vi "workbook.search.vi"(8 "error in":errorcluster, 11 "Client in":refnum<class "Client.lvclass">) -> (0 "error out":errorcluster, 3 "Client out":refnum<class "Client.lvclass">)   [LabVIEW 2020, in "Client.lvclass"]
doc: "Searches for workbooks matching the given filters (text, label, property, asset, or run) and returns a handle list of matches."
uses:
  Client.lvclass
  Client.lvclass/Client.ctl
  client.lvlib
panel:
  out "out_count out":u32
  out "out_list out":i32
  in  "out_list":i32
  in  "asset_rid":string
  in  "property_key":string
  in  "label":string
  in  "search_text":string
  in  "out_count":u32
  in  "run_rid":string
  in  "property_value":string
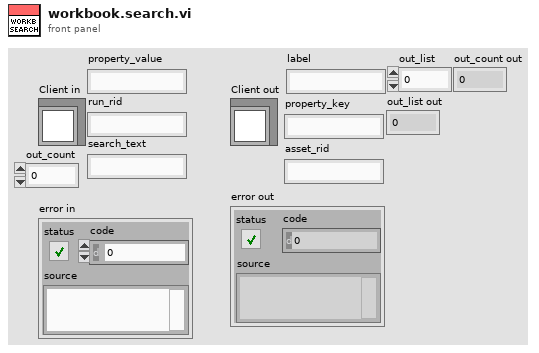
[diagram p1: front panel]
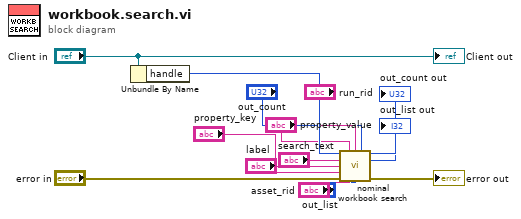
[diagram p0: block diagram]
diagram:
  n1 = Unbundle By Name("Client in") -> ("handle"=w12:i32)
  n2 = call "nominal workbook search.vi"("client"=w12, "property_value"="property_value", "run_rid"="run_rid", "out_count"="out_count", "search_text"="search_text", "label"="label", "property_key"="property_key", "error in (no error)"="error in", "asset_rid"="asset_rid", "out_list"="out_list") -> ("out_list out"=→"out_list out":i32, "out_count out"=→"out_count out":u32, "error out"=→"error out":errorcluster)  [unwired: 2 in, 1 out]
  "Client out" <- "Client in"
